vi "VLCPlayerDemo.vi"() -> ()   [LabVIEW 2015]
uses:
  VLCCommand.ctl
panel:
  out "bytes written":i32
  out "Messages":string
  in  "VLC executable path":path=path "C:/Program Files (x86)/VideoLAN/VLC/vlc.exe"
  in  "Send":bool
  in  "Argument":string
  in  "Command":T1
  in  "stop":bool
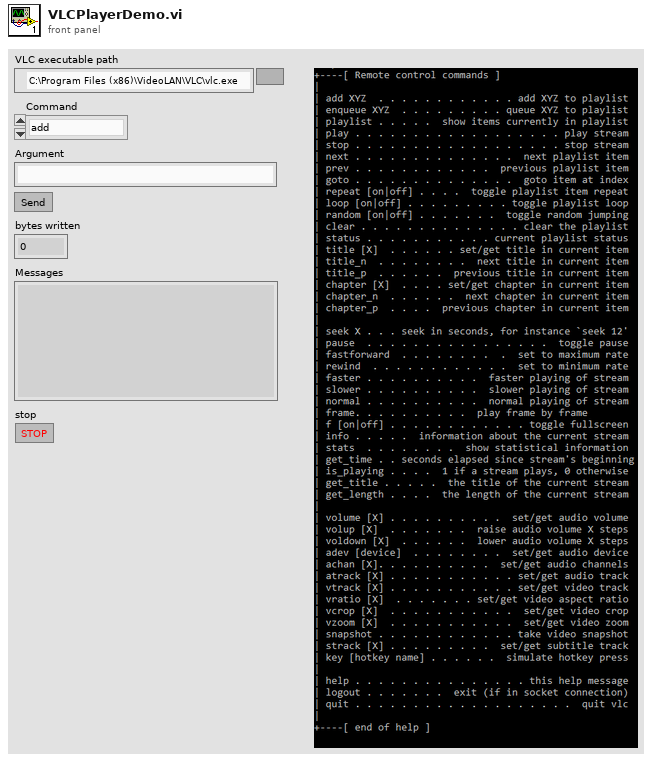
[diagram p1: front panel]
types:
  T1 = typedef "VLCCommand.ctl" = enum16{"add", "enqueue", "playlist", "play", "stop", "next", "prev", "goto", "repeat", "loop", "random", "clear", "status", "title", "title_n", "title_p", "chapter", "chapter_n", "chapter_p", "seek", "pause", "fastforward", "rewind", "faster", "slower", "normal", "frame", "f", "info", "stats", "get_time", "is_playing", "get_title", "get_length", "volume", "volup", "voldown", "adev", "achan", "atrack", "vtrack", "vratio", "vcrop", "vzoom", "snapshot", "strack", "key", "help", "logout", "quit"}
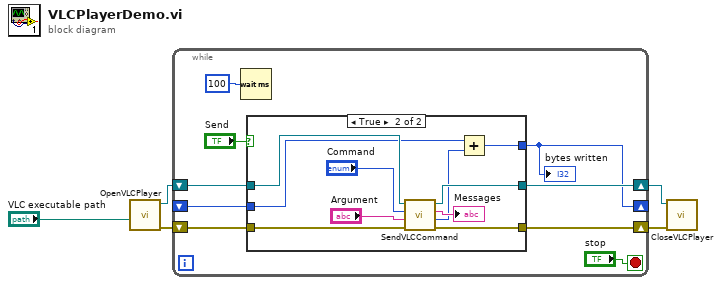
[diagram p0: block diagram]
diagram:
  n1 = call "OpenVLCPlayer.vi"("VLC executable path"="VLC executable path") -> ("error out"=w2:errorcluster, "Connection ID"=w5:refnum<k5>)  [unwired: 9 in]
  n2 = while {
    shift-right: [w13] -> w4
    shift-left: w5 -> [w14]
    shift-right: [w11] -> w1
    shift-left: w2 -> [w12]
    shift-right: [w6] -> _
    shift-left: _ -> [w7]
    stop <- "stop" stop-if-true
    n3 = Wait (ms)(milliseconds to wait=u32 100) -> ()  [unwired: 1 out]
    n4 = case shown="True" "Send" {
      tunnel: w14 -> [w17 w27]
      tunnel: [w17 w26] -> w13
      tunnel: w12 -> [w16 w25]
      tunnel: [w16 w24] -> w11
      tunnel: w7 -> [w15 w19]
      tunnel: [w15 w18] -> w6
      frame False {
      }
      frame True {
        n5 = call "SendVLCCommand.vi"("error in"=w25, "Argument"="Argument", "Command"="Command", "Connection ID in"=w27) -> ("error out"=w24:errorcluster, "bytes written"=w20:i32, "Messages"=→"Messages":string, "Connection ID out"=w26:refnum<k5>)  [unwired: 4 in]
        n6 = Add(x=w19, y=w20) -> (x+y=w18:i32)
      }
    }
    "bytes written" <- w6
  }
  n7 = call "CloseVLCPlayer.vi"("error in"=w1, "Connection ID in"=w4) -> ()  [unwired: 9 in, 1 out]
